vi "APC_9049_HRL_volume.vi"() -> (0 "Volume cluster":T2={"V [m^3]"=[], "dV [m^3/CAD]"=[], "Vdis [m^3]"=0.0, "Surface [m^2]"=[], "CAD/sample"=0.1})   [LabVIEW 2020]
doc: "This VI calculates the cylinder volume information according to the piston position in the cylinder and the crank angle position provided by the CAD vector (the volume matches the the CAD defined as an input, no offset for TDC is considered here)."
uses:
  controls/APC_volume.ctl
panel:
  out "Waveform Graph 2":dbl[](graph)
  in  "Engine cluster":T1={"Lb"=0.217, "Lm"=0.0745, "D"=0.112, "Kc"=12.8, "IVC"=-150.0, "EVO"=150.0, "EVC"=-350.0, "ncyl"=6.0, "offset"=-0.00099}
  out "Waveform Graph":dbl[](graph)
  out "CAD":dbl[](array[numeric])
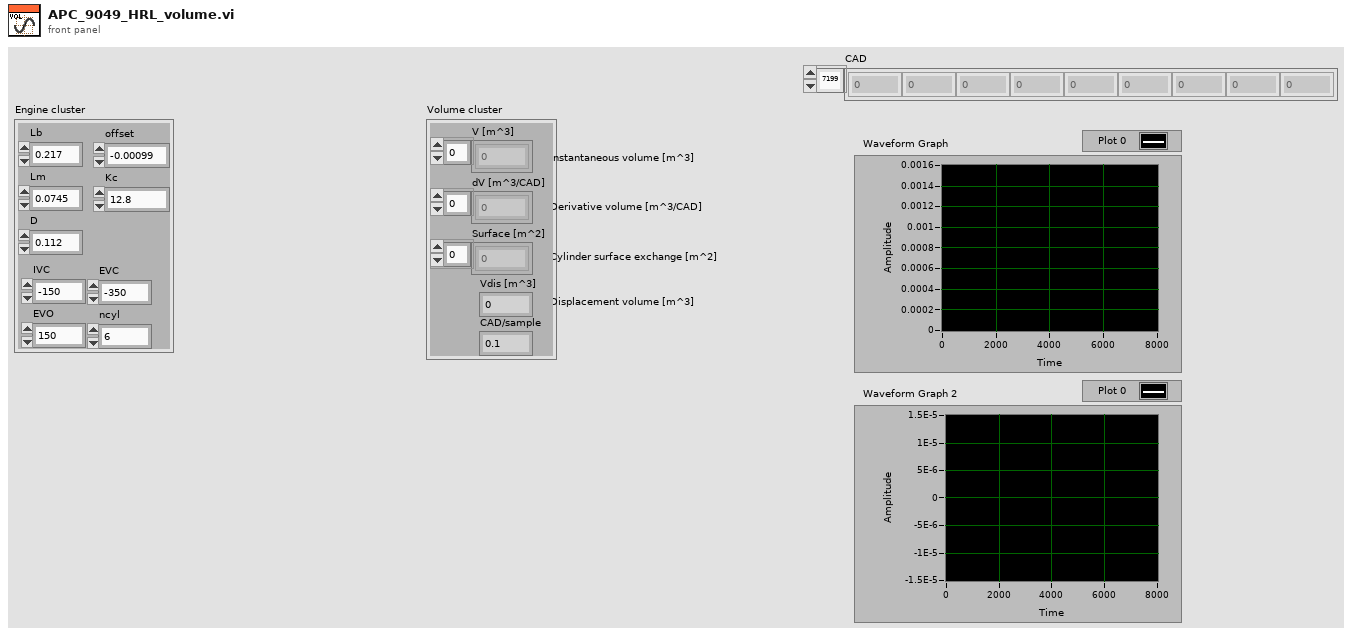
[diagram p1: front panel]
types:
  T1 = cluster{"Lb":dbl, "Lm":dbl, "D":dbl, "Kc":dbl, "IVC":dbl, "EVO":dbl, "EVC":dbl, "ncyl":dbl, "offset":dbl}
  T2 = typedef "APC_volume.ctl" = cluster{"V [m^3]":dbl[], "dV [m^3/CAD]":dbl[], "Vdis [m^3]":dbl, "Surface [m^2]":dbl[], "CAD/sample":dbl}
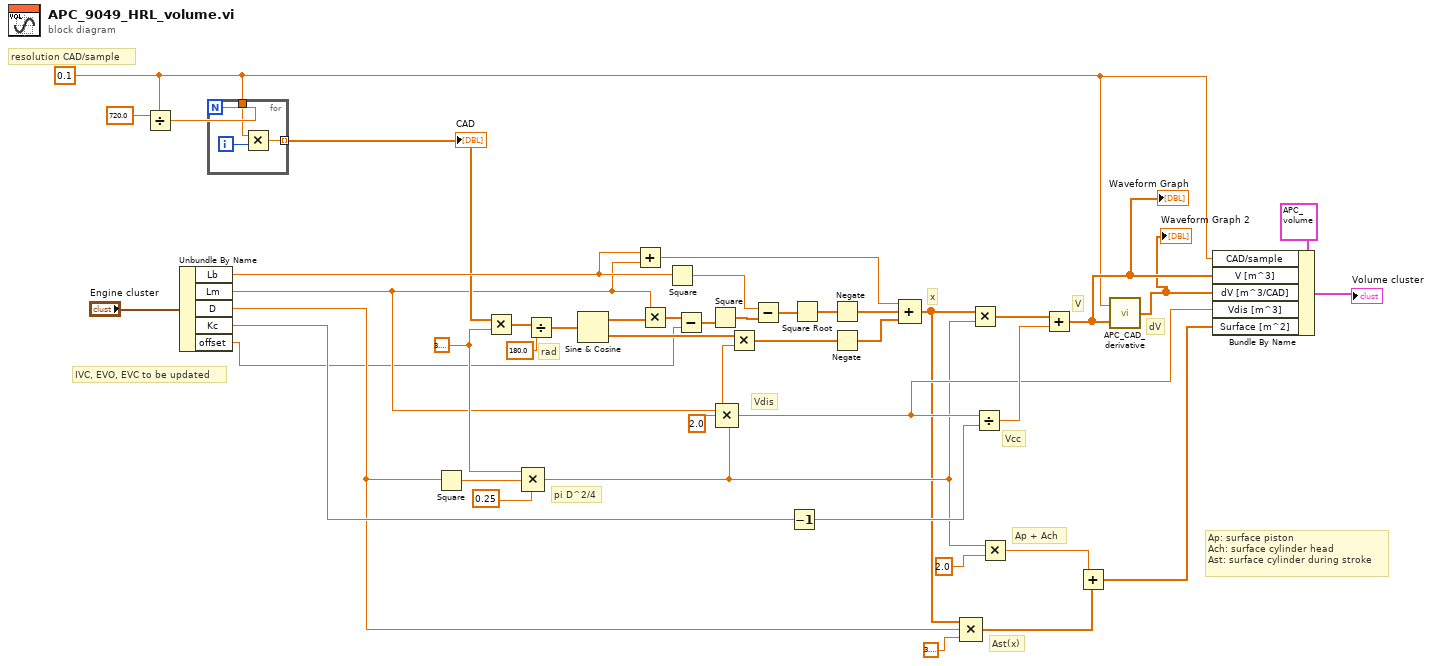
[diagram p0: block diagram]
diagram:
  w1 = 0.1 ("Resolution [CAD/sample]")
  w28 = 3.141592653589793
  # "IVC, EVO, EVC to be updated"
  # "resolution CAD/sample"
  # "rad"
  # "Ast(x)"
  # "Ap: surface piston\nAch: surface cylinder head\nAst: surface cylinder during stroke"
  # "Ap + Ach"
  # "dV"
  # "V"
  # "x"
  # "Vcc"
  # "pi D^2/4"
  # "Vdis"
  n1 = Divide(x=720.0, y=w1) -> (x/y=w13:dbl)
  n2 = Unbundle By Name("Engine cluster") -> ("Lb"=w27:dbl, "Lm"=w9:dbl, "D"=w20:dbl, "Kc"=w32:dbl, "offset"=w5:dbl)
  n3 = for {
    N: w13 -> [_]
    tunnel: w1 -> [w47]
    tunnel: [w46] -> w12 mode=indexing
    i -> [w45]
    n4 = Multiply(x=w47, y=w45) -> (x*y=w46:dbl)
  }
  "CAD" <- w12
  n5 = Square(x=w20) -> (x^2=w36:dbl)
  n6 = Multiply(x=w12, y=w28) -> (x*y=w44:dbl[])
  n7 = Compound Arithmetic op=MULTIPLY(w28, w36, 0.25 ("value")) -> (w23:dbl)
  n8 = Divide(x=w44, y=180.0) -> (x/y=w43:dbl[])
  n9 = Sine & Cosine(0:w43) -> (1:w8:dbl[], 2:w29:dbl[])
  n10 = Add(x=w27, y=w9) -> (x+y=w26:dbl)
  n11 = Multiply(x=w9, y=w8) -> (x*y=w7:dbl[])
  n12 = Square(x=w27) -> (x^2=w42:dbl)
  n13 = Subtract(x=w7, y=w5) -> (x-y=w6:dbl[])
  n14 = Square(x=w6) -> (x^2=w10:dbl[])
  n15 = Compound Arithmetic op=MULTIPLY(w9, 2.0 ("value"), w23) -> (w24:dbl)
  n16 = Multiply(x=w29, y=w9) -> (x*y=w39:dbl[])
  n17 = Subtract(x=w42, y=w10) -> (x-y=w41:dbl[])
  n18 = Decrement(x=w32) -> (x-1=w25:dbl)
  n19 = Square Root(x=w41) -> (sqrt(x)=w40:dbl[])
  n20 = Negate(x=w40) -> (-x=w37:dbl[])
  n21 = Negate(x=w39) -> (-x=w38:dbl[])
  n22 = Compound Arithmetic op=ADD(w26, w37, w38) -> (w19:dbl[])
  n23 = Compound Arithmetic op=MULTIPLY(w19, w20, 3.141592653589793) -> (w18:dbl[])
  n24 = Multiply(x=w19, y=w23) -> (x*y=w34:dbl[])
  n25 = Divide(x=w24, y=w25) -> (x/y=w33:dbl)
  n26 = Multiply(x=w23, y=2.0) -> (x*y=w17:dbl)
  n27 = Add(x=w34, y=w33) -> (x+y=w11:dbl[])
  "Waveform Graph" <- w11
  n28 = Add(x=w17, y=w18) -> (x+y=w16:dbl[])
  n29 = call "APC_CAD_derivative.vi"("x (e.g., pcyl)"=w11, "Encoder res. [CAD/sample]"=w1) -> ("dx/dCAD"=w4:dbl[])
  "Waveform Graph 2" <- w4
  n30 = Bundle By Name(cluster=T2 {"V [m^3]"=array[7200 elements], "dV [m^3/CAD]"=array[7200 elements], "Vdis [m^3]"=0.0014679531496869813, "Surface [m^2]"=array[7200 elements], "CAD/sample"=0.1} ("Volume cluster"), "CAD/sample"=w1, "V [m^3]"=w11, "dV [m^3/CAD]"=w4, "Vdis [m^3]"=w24, "Surface [m^2]"=w16) -> (→"Volume cluster":T2)
